vi "Test Waveguide Model.vi"() -> ()   [LabVIEW 2019, in "Instrument.Lockin.lvlib" / "Instrument.DAQ.lvclass"]
uses:
  Instrument.DAQ.lvclass
  330ec20b-b548-4883-a0db-27ae69a953e4.vi
  4bca89b2-e569-4c1e-b6e4-4a556962b757.vi
  b5ca3f61-d14b-46d2-bb90-c1bf30874911.vi
  <vilib>/Analysis/NI_AALBase.lvlib
panel:
  out "Waveform Graph from VIM":dbl[](graph)
  out "Waveform Graph":dbl[](graph)
  in  "Vsg step (V)":dbl=0.001 format="%#_6p"
  in  "Vsg end (V)":dbl=0.1 format="%#_6p"
  in  "Vsg start (V)":dbl format="%#_6p"
  out "I vs Vsg":cluster{dbl[], dbl[]}(graph)
  in  "V_source (V)":dbl=0.001 format="%#_6p"
  out "G vs Vsg":cluster{dbl[], dbl[]}(graph)
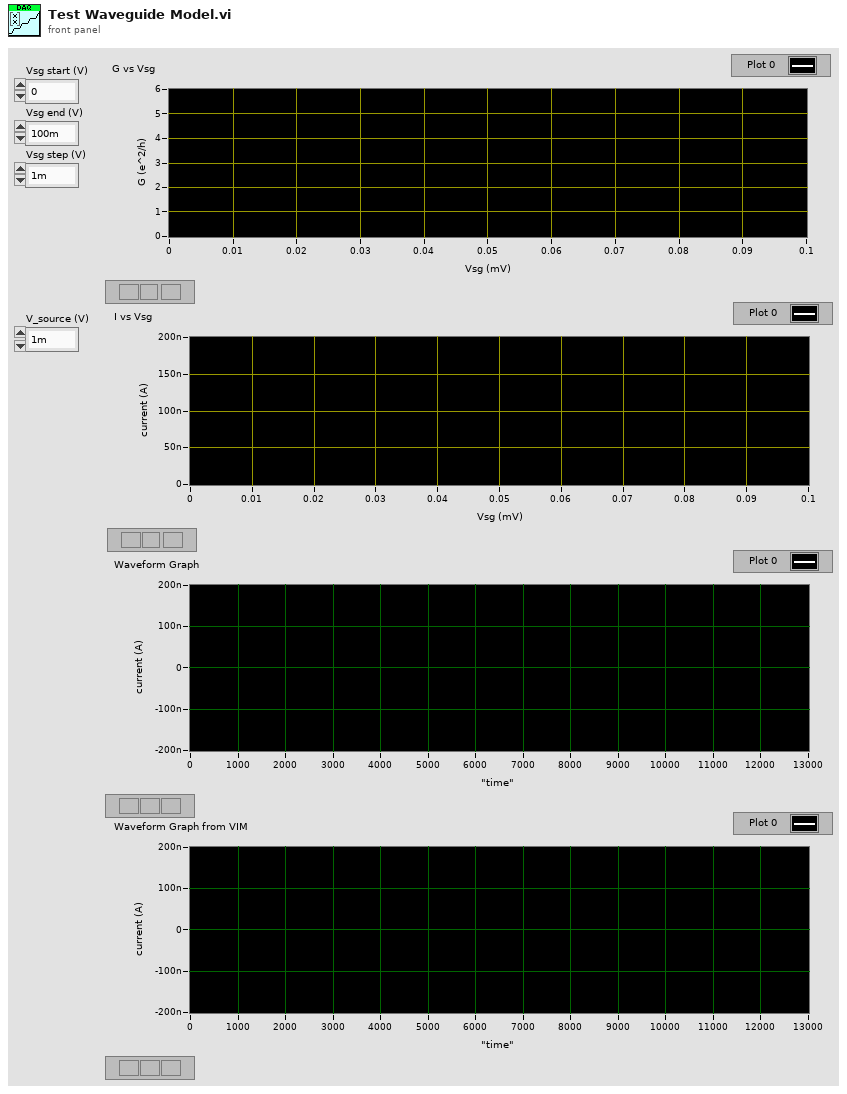
[diagram p1: front panel]
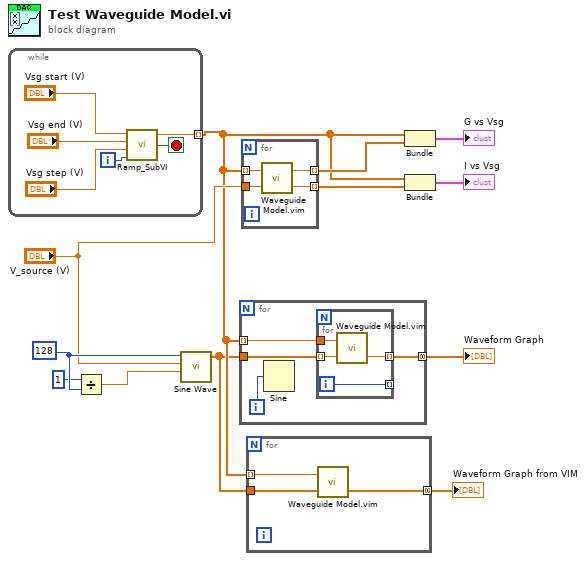
[diagram p0: block diagram]
diagram:
  w7 = 128 ("samples")
  n1 = while {
    tunnel: [w18] -> w3 mode=indexing
    i -> [w14]
    stop <- w13 stop-if-true
    n2 = call <userlib>:"Ramp_SubVI.vi"("index"=w14, "step"="Vsg step (V)", "end"="Vsg end (V)", "start"="Vsg start (V)") -> ("Stop?"=w13:bool, "Numeric"=w18:dbl)  [unwired: 1 in]
  }
  n3 = Divide(x=1, y=w7) -> (x/y=w5:dbl)
  n4 = call <vilib>:"Sine Wave.vi"("samples"=w7, "amplitude"="V_source (V)", "frequency"=w5) -> ("sine wave"=w2:dbl[])  [unwired: 2 in, 2 out]
  n5 = for {
    tunnel: w2 -> [w22]
    tunnel: [w21] -> w8 mode=concatenating
    tunnel: w3 -> [w20] mode=indexing
    i -> [w19]
    n6 = Sine(x=w19) -> ()  [unwired: 1 out]
    n7 = for {
      tunnel: w22 -> [w26] mode=indexing
      tunnel: [w25] -> w21 mode=indexing
      tunnel: [w24] -> _ mode=indexing
      tunnel: w20 -> [w23]
      i -> [w24]
      n8 = call "Waveguide Model.vim"("Vs (V)"=w26, "Vsg (V)"=w23) -> ("I[Vsg] (A)"=w25:dbl)  [unwired: 1 out]
    }
  }
  "Waveform Graph" <- w8
  n9 = for {
    tunnel: w3 -> [w30] mode=indexing
    tunnel: [w28] -> w9 mode=indexing
    tunnel: "V_source (V)" -> [w29]
    tunnel: [w27] -> w10 mode=indexing
    n10 = call "Waveguide Model.vim"("Vs (V)"=w29, "Vsg (V)"=w30) -> ("I[Vsg] (A)"=w27:dbl, "G[Vsg] (e2/h)"=w28:dbl)
  }
  n11 = for {
    tunnel: w3 -> [w33] mode=indexing
    tunnel: w2 -> [w32]
    tunnel: [w31] -> w1 mode=concatenating
    n12 = call "Waveguide Model.vim"("Vs (V)"=w32, "Vsg (V)"=w33) -> ("I[Vsg] (A)"=w31:dbl[])  [unwired: 1 out]
  }
  "Waveform Graph from VIM" <- w1
  n13 = Bundle(w3, w9) -> (→"G vs Vsg":cluster{dbl[], dbl[]})  [unwired: 1 in]
  n14 = Bundle(w3, w10) -> (→"I vs Vsg":cluster{dbl[], dbl[]})  [unwired: 1 in]
